vi "niRFUtil MT UTIL Apply Frequency Offset (Complex SGL).vi"(0 "Signal In":T1 format="%.2f", 5 "sine":dbl, 7 "cosine":dbl, 9 "real (phasor) in":cdb) -> (4 "Signal Out":T1 format="%.2f", 6 "phasor out":cdb)   [LabVIEW 2015, in "niRFUtil.lvlib"]
uses:
  niRFUtil.lvlib
  Includes/niRFUtil INC Complex Array.ctl
  niRFDMT.dll
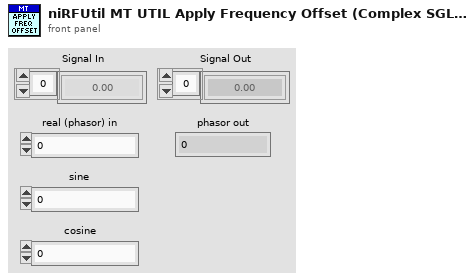
[diagram p1: front panel]
types:
  T1 = typedef "niRFUtil.lvlib/niRFUtil INC Complex Array.ctl" = csg[]
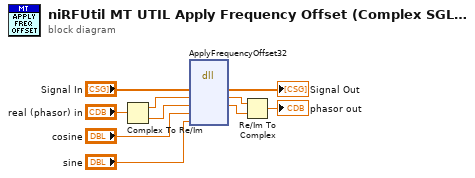
[diagram p0: block diagram]
diagram:
  n1 = Complex To Re/Im(x + iy="real (phasor) in") -> (x=w5:dbl, y=w4:dbl)
  n2 = dll-call lib="C:/Perforce/semoore-sales/Customers/NATI-3813/Noise Floor/LV Filters/ParallelComplexFilterRFUtil/niRFUtil/MT/Utilities/niRFDMT.*" fn="ApplyFrequencyOffset32"("samples"="Signal In", "real_phasor"=w5, "imag_phasor"=w4, "cosine"="cosine", "sine"="sine") -> ("samples"=→"Signal Out":T1, "real_phasor"=w3:dbl, "imag_phasor"=w2:dbl)  [unwired: 5 in, 3 out]
  n3 = Re/Im To Complex(1:w2, 2:w3) -> (0:→"phasor out":cdb)
